vi "SD Read Name Cache.vi"(10 "Name":string, 11 "Table Prefix":string="SmartDashboard") -> (2 "Success":bool, 3 "Field Value Out":T1)   [LabVIEW 2017]
uses:
  <vilib>/Rock Robotics/Network Tables/Field Data.ctl
  <vilib>/Rock Robotics/Network Tables/Field Type.ctl
  <vilib>/Rock Robotics/Network Tables/Sequence.ctl
  <vilib>/Rock Robotics/Network Tables/Make Table Operation.ctl
  <vilib>/Rock Robotics/Network Tables/NT Globals.vi
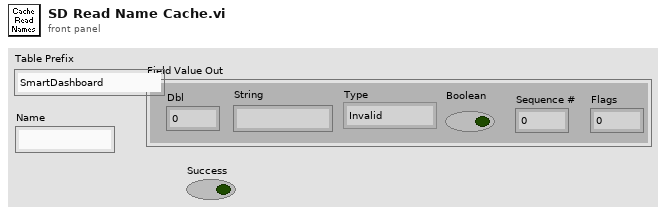
[diagram p1: front panel]
types:
  T1 = typedef "Field Data.ctl" = cluster{"Dbl":dbl, "String":string, "Type":T2, "Boolean":bool, "Sequence #":T3, "Flags":u8}
  T2 = typedef "Field Type.ctl" = enum8{"Invalid", "Bool", "Numeric", "String", "Raw", "Boolean Array", "Numeric Array", "String Array", "RPC"}
  T3 = typedef "Sequence.ctl" = u16
  T4 = typedef "Make Table Operation.ctl" = enum16{"Get or Add Field", "Get Field or Add Temp", "Replace Temp ID", "Get Field ID - No Add", "Get Table Field IDs", "Get Field ID Info", "Move Field to Temp", "Validate", "Remove Field", "Remove All"}
  T5 = typedef "Field ID.ctl" = i32
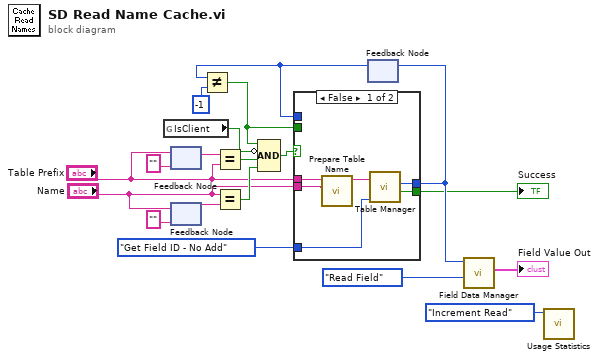
[diagram p0: block diagram]
diagram:
  n1 = global read "NT Globals.vi" "IsClient"() -> (w16:bool)
  n2 = feedback #1("" ("Name")) -> (w15:string)
  n3 = feedback-in #1("Table Prefix") -> ()
  n4 = feedback #2("" ("Name")) -> (w4:string)
  n5 = feedback-in #2("Name") -> ()
  n6 = Equal?(x=w15, y="Table Prefix") -> (x = y?=w17:bool)
  n7 = Equal?(x="Name", y=w4) -> (x = y?=w3:bool)
  n8 = feedback #3() -> (w8:T5)  [unwired: 1 in]
  n9 = Not Equal?(x=w8, y=-1) -> (x != y?=w7:bool)
  n10 = Compound Arithmetic op=AND(w7, invert w16, w17, w3) -> (w18:bool)
  n11 = case shown="False" w18 {
    tunnel: "Table Prefix" -> [w20 _]
    tunnel: [w25 w27] -> w12
    tunnel: [w24 w26] -> w11
    tunnel: Make_Table_Operation."Get Field ID - No Add" ("Operation") -> [w23 _]
    tunnel: w8 -> [_ w27]
    tunnel: w7 -> [_ w26]
    tunnel: "Name" -> [w21 _]
    frame False {
      n12 = call <vilib>:"Prepare Table Name.vi"("Name"=w21, "Table Prefix"=w20) -> ("Prefixed Name"=w22:string)  [unwired: 9 in]
      n13 = call <vilib>:"Table Manager.vi"("Operation"=w23, "Entry Name"=w22) -> ("Success"=w24:bool, "Entry ID"=w25:T5)  [unwired: 6 in, 2 out]
    }
    frame True {
    }
  }
  "Success" <- w11
  n14 = feedback-in #3(w12) -> ()
  n15 = call <vilib>:"Field Data Manager.vi"("Operation"=enum16{"Update Field", "Read Field"}."Read Field", "Field ID"=w12) -> ("Field Value Out"=→"Field Value Out":T1)  [unwired: 8 in, 1 out]
  n16 = call <vilib>:"Usage Statistics.vi"("Operation"=enum16{"Increment Read", "Increment Write"}."Increment Read") -> ()  [unwired: 11 in]
